vi "Receive.vi"(10 "Msg Strategy in":refnum<class "Msg Strategy.lvclass">, 11 "Base Event in":refnum<class "Base Event.lvclass">) -> (2 "Msg Strategy out":refnum<class "Msg Strategy.lvclass">, 3 "Base Event out":refnum<class "Base Event.lvclass">)   [LabVIEW 2021, in "jettl.lvlib" / "Base Event.lvlib" / "Base Event.lvclass"]
uses:
  Base Event.lvclass
  Msg Strategy/Msg Strategy.lvclass
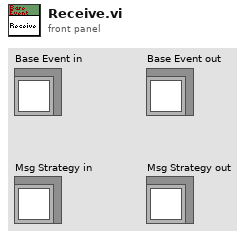
[diagram p1: front panel]
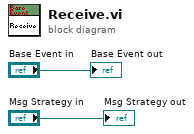
[diagram p0: block diagram]
diagram:
  "Base Event out" <- "Base Event in"
  "Msg Strategy out" <- "Msg Strategy in"
